vi "Parse Action State After Exit.vi"(11 "States":string) -> (1 "Need to Process":string, 3 "Remaining States":string)   [LabVIEW 2017, in "CSM Shared.lvlib"]
uses:
  CSM Shared.lvlib
  Trim Single-line Text.vi
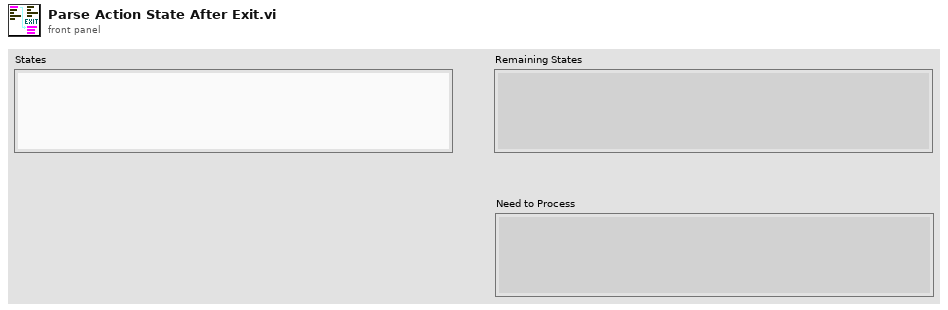
[diagram p1: front panel]
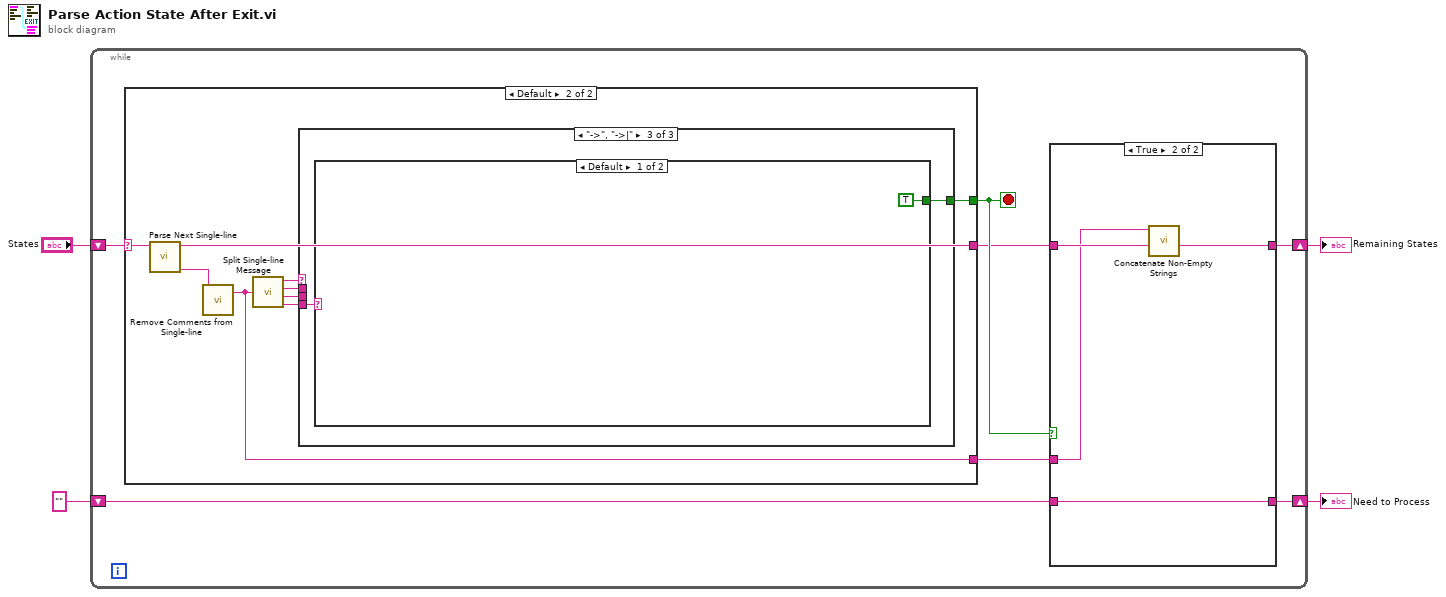
[diagram p0: block diagram]
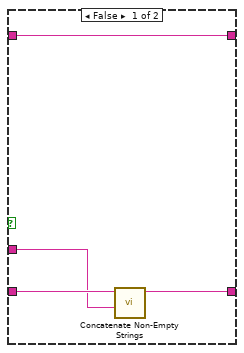
[diagram p2: hidden frame]
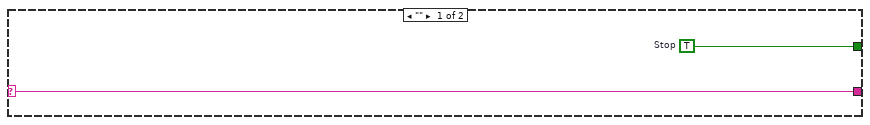
[diagram p3: hidden frame]
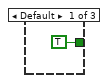
[diagram p4: hidden frame]
diagram:
  n1 = while {
    shift-right: [w6] -> w3
    shift-left: "States" -> [w11]
    shift-right: [w10] -> w1
    shift-left: "" ("States 2") -> [w9]
    stop <- w7 stop-if-true
    n2 = case shown="Default" w11 {
      selector: w11 -> [w20 w30]
      tunnel: [w20 w24] -> w5
      tunnel: [w21 w23] -> w7
      tunnel: [_ w22] -> w8
      frame "" {
        w21 = TRUE  # Stop
      }
      frame Default {
        n3 = call "Parse Next Single-line.vi"("States Queue"=w30) -> ("Next Single-line State"=w25:string, "Remaining States Queue"=w24:string)  [unwired: 9 in]
        n4 = call "Remove Comments from Single-line.vi"("single-line text"=w25) -> ("single-line text without comments"=w22:string)  [unwired: 2 in]
        n5 = call "Split Single-line Message.vi"("single-line text"=w22) -> ("operator"=w26:string, "state"=w29:string, "args"=w28:string, "source/target"=w27:string)  [unwired: 6 in]
        n6 = case shown="\"->\", \"->|\"" w26 {
          tunnel: w28 -> [_ _ _]
          tunnel: w27 -> [_ _ w33]
          tunnel: w29 -> [_ _ _]
          tunnel: [TRUE ("Internal State(-&)") _ w32] -> w23
          frame Default {
          }
          frame "-&" {
          }
          frame "->", "->|" {
            n7 = case shown="Default" w33 {
              tunnel: [TRUE ("Internal State(-&)") _] -> w32
              frame Default {
              }
              frame "<all>", "<broadcast>", "<interput>", "<interrupt>", "<interupt>", "<state>", "<status>" {
              }
            }
          }
        }
      }
    }
    n8 = case shown="True" w7 {
      tunnel: [w14 w19] -> w10
      tunnel: w9 -> [w13 w19]
      tunnel: w8 -> [w12 w17]
      tunnel: [w15 w16] -> w6
      tunnel: w5 -> [w15 w18]
      frame False {
        n9 = call "Concatenate Non-Empty Strings.vi"("String2"=w12, "String1"=w13) -> ("Result String"=w14:string)  [unwired: 6 in]
      }
      frame True {
        n10 = call "Concatenate Non-Empty Strings.vi"("String2"=w18, "String1"=w17) -> ("Result String"=w16:string)  [unwired: 6 in]
      }
    }
  }
  "Remaining States" <- w3
  "Need to Process" <- w1
